vi "Set the Impedancel According to Range in Autosetup_FP-Scope SP.vi"(7 "BandWidth":dbl) -> (8 "BandWidth":i32)   [LabVIEW 2012]
doc: "根据自动调整后的BandWidth获取BandWidth下拉列表的值"
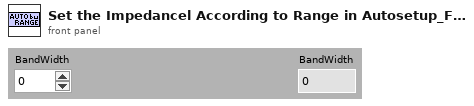
[diagram p1: front panel]
types:
  T1 = typedef "INI Properties_DStr-Scope SP.ctl" = cluster{"Channels":cluster{"String":string, "Value":ext}[], "VoltInterval":cluster{"String":string, "Value":ext}[], "Impedance":cluster{"String":string, "Value":ext}[], "Bandwidth":cluster{"String":string, "Value":ext}[], "TimeInterval":cluster{"String":string, "Value":ext}[], "Type":cluster{"String":string, "Value":ext}[], "Source":cluster{"String":string, "Value":ext}[], "DigiSource":cluster{"String":string, "Value":ext}[], "TrigCpl":cluster{"String":string, "Value":ext}[], "EXTCpl":cluster{"String":string, "Value":ext}[], "Mode":cluster{"String":string, "Value":ext}[], "Event":cluster{"String":string, "Value":ext}[], "Format":cluster{"String":string, "Value":ext}[], "OffsetVisible":bool[], "Offset":dbl[][], "Point":dbl[][], "TrigLev":dbl[][], "Win":dbl[][], "Leve":dbl[][], "ExtLev":dbl[][], "PolaEnable":u8, "RISEnable":u8, "ChanCpl":cluster{"String":string, "Value":ext}[], "TimeValue":dbl[], "VoltValue":dbl[], "ImpedanceValue":dbl[], "BandwidthValue":dbl[]}
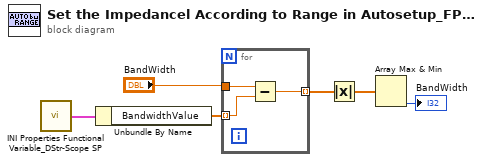
[diagram p0: block diagram]
diagram:
  n1 = call "INI Properties Functional Variable_DStr-Scope SP.vi"() -> ("proper"=w3:T1)  [unwired: 15 in]
  n2 = Unbundle By Name(w3) -> ("BandwidthValue"=w2:dbl[])
  n3 = for {
    tunnel: w2 -> [w8] mode=indexing
    tunnel: "BandWidth" -> [w9]
    tunnel: [w7] -> w6 mode=indexing
    n4 = Subtract(x=w9, y=w8) -> (x-y=w7:dbl)
  }
  n5 = Absolute Value(x=w6) -> (abs(x)=w5:dbl[])
  n6 = Array Max & Min(array=w5) -> (min index (indices)=→"BandWidth":i32)  [unwired: 3 out]
